vi "ProSCI DebugGlobal.vi"() -> ()   [LabVIEW 2012]
panel:
  out "gDbgRobotWait":u32
  out "gDebug":string
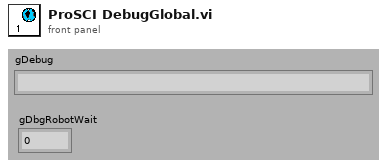
[diagram p1: front panel]
diagram:
